vi "Timed Button Press Updated.vi"(10 "Holdtime (ms)":u32, 11 "Input":bool) -> (0 "Press?":bool, 1 "Long Press Held":bool, 2 "Long Press":bool, 3 "Quick Press":bool)   [LabVIEW 2019]
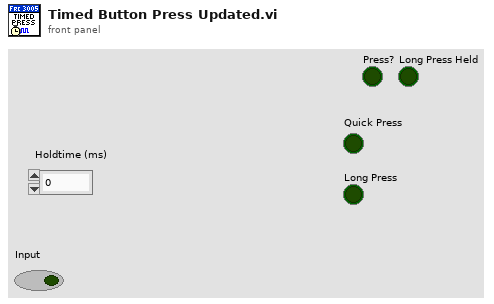
[diagram p1: front panel]
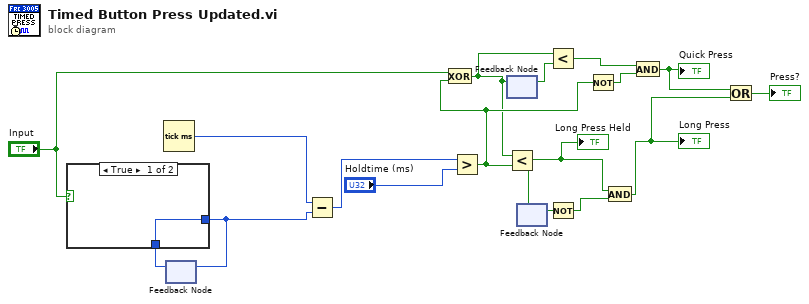
[diagram p0: block diagram]
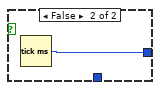
[diagram p2: hidden frame]
diagram:
  n1 = Tick Count (ms)() -> (millisecond timer value=w8:u32)
  n2 = feedback #1() -> (w5:u32)  [unwired: 1 in]
  n3 = case shown="True" "Input" {
    tunnel: [w18 w19] -> w6
    tunnel: w5 -> [w18 _]
    frame True {
    }
    frame False {
      n4 = Tick Count (ms)() -> (millisecond timer value=w19:u32)
    }
  }
  n5 = feedback-in #1(w6) -> ()
  n6 = Subtract(x=w8, y=w6) -> (x-y=w7:u32)
  n7 = Greater?(x=w7, y="Holdtime (ms)") -> (0:w17:bool)
  n8 = Exclusive Or(1:w17, 2:"Input") -> (0:w14:bool)
  n9 = feedback #2() -> (w12:bool)  [unwired: 1 in]
  n10 = feedback-in #2(w14) -> ()
  n11 = Less?(x=w14, y=w17) -> (x < y?=w13:bool)
  "Long Press Held" <- w13
  n12 = feedback #3() -> (w10:bool)  [unwired: 1 in]
  n13 = feedback-in #3(w13) -> ()
  n14 = Less?(x=w14, y=w12) -> (x < y?=w15:bool)
  n15 = Not(x=w10) -> (.not. x?=w11:bool)
  n16 = Not(x=w17) -> (.not. x?=w16:bool)
  n17 = And(x=w13, y=w11) -> (x .and. y?=w3:bool)
  "Long Press" <- w3
  n18 = And(x=w15, y=w16) -> (x .and. y?=w4:bool)
  "Quick Press" <- w4
  n19 = Or(x=w4, y=w3) -> (x .or. y?=→"Press?":bool)
